vi "ConvertSensorRatioToSensitivity.vi"(11 "sensor ratio":string) -> (3 "sensitivity":dbl)   [LabVIEW 2017, in "McsaFpgaAcquisition.lvlib"]
uses:
  <vilib>/addons/InsightCM/Devices/Shared/Mcsa/McsaFpgaAcquisition/McsaFpgaAcquisition.lvlib
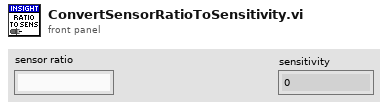
[diagram p1: front panel]
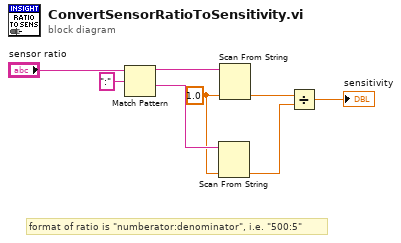
[diagram p0: block diagram]
diagram:
  w4 = 1.0 ("default value 1")
  # "format of ratio is \"numberator:denominator\", i.e. \"500:5\""
  n1 = Match Pattern(string="sensor ratio", regular expression=":") -> (before substring=w6:string, after substring=w5:string)  [unwired: 1 in, 2 out]
  n2 = Scan From String(input string=w5, default 1=w4) -> (output 1=w2:dbl)  [unwired: 3 in, 3 out]
  n3 = Scan From String(input string=w6, default 1=w4) -> (output 1=w3:dbl)  [unwired: 3 in, 3 out]
  n4 = Divide(x=w3, y=w2) -> (x/y=→"sensitivity":dbl)
